vi "Init Hardware.vi"(8 "error in (no error)":errorcluster, 11 "Tektronix MSO 6 Driver in":refnum<class "Tektronix MSO 6 Driver.lvclass">) -> (0 "error out":errorcluster, 3 "Tektronix MSO 6 Driver out":refnum<class "Tektronix MSO 6 Driver.lvclass">)   [LabVIEW 2021, in "Tektronix MSO 6 Driver.lvclass"]
uses:
  Tektronix MSO 6 Driver.lvclass
  C:/GitHub/NHMFL_Core/Libraries/Instruments/Tektronix/Tektronix Driver/Tektronix Driver.lvclass
  C:/GitHub/NHMFL_Core/Libraries/Instruments/Instrument Driver/Instrument Driver.lvclass
  Instrument Driver/Instrument Driver.lvclass/Instrument Driver.ctl
  Instrument Driver/Write Group name.vi
  Instrument Driver/Write Channel names.vi
  <instrlib>/Tektronix MSO5X Series/Public/Configure/Configure Trigger (Edge).vi
  Tektronix MSO 6 Driver.lvclass/Tektronix MSO 6 Driver.ctl
  <instrlib>/Tektronix MSO5X Series/Tektronix MSO5X Series.lvlib
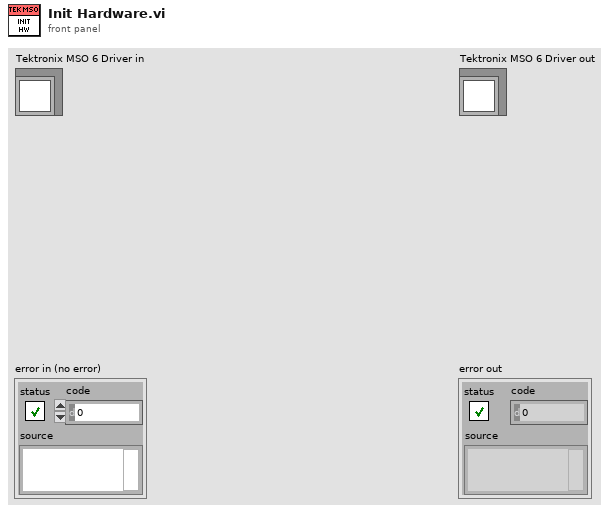
[diagram p1: front panel]
types:
  T1 = typedef "Tektronix Configuration.ctl" = cluster{"Channel":i32, "Number of averages":i32, "Input impedace":enum16{"1 M Ohm", "50 Ohm"}, "Vertical coupling":enum16{"AC", "DC", "Ground"}}
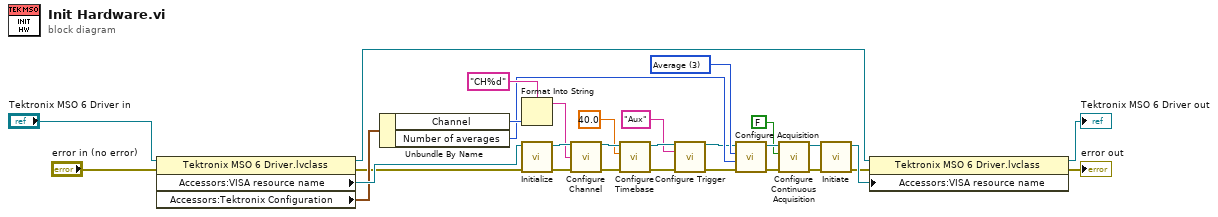
[diagram p0: block diagram]
diagram:
  w24 = u16 3 items=["Sample", "Peak Detect", "Hi Res", "Average", "Envelope"] ("Acquisition Type (0:Sample)")
  n1 = property class="Tektronix MSO 6 Driver.lvclass"(reference="Tektronix MSO 6 Driver in", error in="error in (no error)") -> (reference out=w19:refnum<class "Tektronix MSO 6 Driver.lvclass">, error out=w23:errorcluster, "Accessors:VISA resource name"=w29:refnum<visa-resource-name>, "Accessors:Tektronix Configuration"=w28:T1)
  n2 = Unbundle By Name(w28) -> ("Channel"=w27:i32, "Number of averages"=w25:i32)
  n3 = Format Into String(format string="CH%d", w27) -> (resulting string=w1:string)  [unwired: 2 in, 1 out]
  n4 = call <instrlib>:"Initialize.vi"("error in (no error)"=w23, "VISA resource name"=w29) -> ("error out"=w20:errorcluster, "VISA resource name out"=w21:refnum<visa-resource-name>)  [unwired: 8 in]
  n5 = call <instrlib>:"Configure Channel.vi"("VISA resource name"=w21, "Channel (CH1)"=w1, "error in (no error)"=w20) -> ("VISA resource name out"=w11:refnum<visa-resource-name>, "error out"=w8:errorcluster)  [unwired: 11 in]
  n6 = call <instrlib>:"Configure Timebase.vi"("error in (no error)"=w8, "Timebase (40 ns)"=40.0, "VISA resource name"=w11) -> ("error out"=w12:errorcluster, "VISA resource name out"=w13:refnum<visa-resource-name>)  [unwired: 7 in]
  n7 = call-poly <instrlib>:"Configure Trigger.vi"("VISA resource name"=w13, "Trigger Source (CH1)"="Aux", "error in (no error)"=w12) -> ("VISA resource name out"=w10:refnum<visa-resource-name>, "error out"=w7:errorcluster)  [unwired: 11 in]
  n8 = call <instrlib>:"Configure Acquisition.vi"("error in (no error)"=w7, "Average Waveforms (16)"=w25, "Acquisition Type (0:Sample)"=w24, "VISA resource name"=w10) -> ("error out"=w14:errorcluster, "VISA resource name out"=w16:refnum<visa-resource-name>)  [unwired: 6 in]
  n9 = call <instrlib>:"Configure Continuous Acquisition.vi"("error in (no error)"=w14, "Enable Continuous Acquisition Mode (True)"=FALSE, "VISA resource name"=w16) -> ("error out"=w3:errorcluster, "VISA resource name out"=w5:refnum<visa-resource-name>)  [unwired: 7 in]
  n10 = call <instrlib>:"Initiate.vi"("error in (no error)"=w3, "VISA resource name"=w5) -> ("error out"=w2:errorcluster, "VISA resource name out"=w4:refnum<visa-resource-name>)  [unwired: 8 in]
  n11 = property class="Tektronix MSO 6 Driver.lvclass"(reference=w19, error in=w2, "Accessors:VISA resource name"=w4) -> (reference out=→"Tektronix MSO 6 Driver out":refnum<class "Tektronix MSO 6 Driver.lvclass">, error out=→"error out":errorcluster)
